vi "Define Events.vi"(8 "error in (no error)":errorcluster, 11 "Example Source in":refnum<class "Example Source.lvclass">) -> (0 "error out":errorcluster, 3 "Example Source out":refnum<class "Example Source.lvclass">)   [LabVIEW 2016, in "Example Source.lvlib" / "Example Source.lvclass"]
doc: "This dynamic dispatch VI has to be overriden by the concrete Souce Actor subclasses in order to define the event served by the source"
uses:
  Example Source.lvclass
  C:/Projects/Shared Libraries/Event Actors/Event Source/Event Source.lvclass
  Example Events/Double Array Event.lvclass
  C:/Projects/Shared Libraries/Event Actors/Event/Event.lvclass
  Example Events/Timestamp Event.lvclass
  Example Events/Boolean Event.lvclass
  Event/Event.lvclass/Event.ctl
  Event/Event.lvclass
  Event Source/Event Source.lvclass
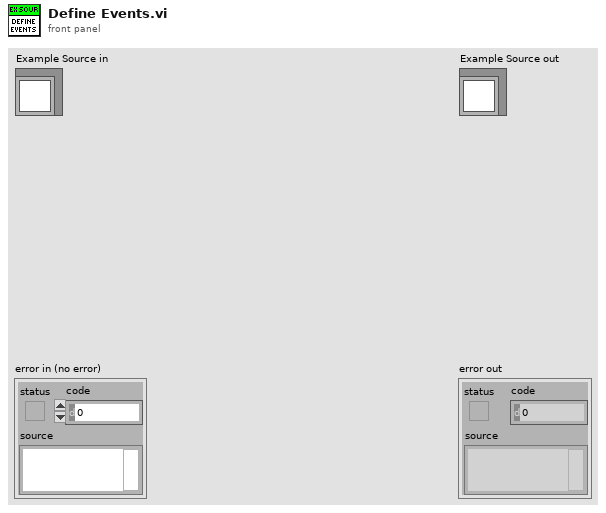
[diagram p1: front panel]
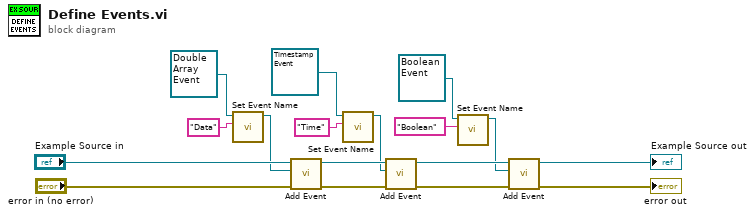
[diagram p0: block diagram]
diagram:
  n1 = call "Set Event Name.vi"("Name (Generic)"="Data", "Event In"=refnum<class "Double Array Event.lvclass"> refnum ("Double Array Event.lvclass")) -> ("Event Out"=w8:refnum<class "Double Array Event.lvclass">)  [unwired: 9 in]
  n2 = call "Add Event.vi"("error in (no error)"="error in (no error)", "Event"=w8, "Event Source in"="Example Source in") -> ("error out"=w4:errorcluster, "Event Source out"=w10:refnum<class "Example Source.lvclass">)  [unwired: 7 in]
  n3 = call "Set Event Name.vi"("Name (Generic)"="Time", "Event In"=refnum<class "Timestamp Event.lvclass"> refnum ("Timestamp Event.lvclass")) -> ("Event Out"=w7:refnum<class "Timestamp Event.lvclass">)  [unwired: 9 in]
  n4 = call "Add Event.vi"("error in (no error)"=w4, "Event"=w7, "Event Source in"=w10) -> ("error out"=w3:errorcluster, "Event Source out"=w9:refnum<class "Example Source.lvclass">)  [unwired: 7 in]
  n5 = call "Set Event Name.vi"("Name (Generic)"="Boolean", "Event In"=refnum<class "Boolean Event.lvclass"> refnum ("Example Source.lvlib:Boolean Event.lvclass")) -> ("Event Out"=w6:refnum<class "Boolean Event.lvclass">)  [unwired: 9 in]
  n6 = call "Add Event.vi"("error in (no error)"=w3, "Event"=w6, "Event Source in"=w9) -> ("error out"=→"error out":errorcluster, "Event Source out"=→"Example Source out":refnum<class "Example Source.lvclass">)  [unwired: 7 in]
